vi "Test Executive.vi"(11 "Module Config":T30={"Name"="Test Executive", "Parent Q"=refnum, "Is Child?"=FALSE, "Index"=0, "Dirs"={"Root"=path "C:/MTE", "Config"=path "C:/MTE/Config", "Logs"=path "C:/MTE/Logs", "Reports"=path "C:/ATE/Reports", "App Data"=path "C:/ProgramData/Test Executive"}, "Simulate"=FALSE, "SimCtrl"=refnum}) -> ()   [LabVIEW 2018] (continued)
          frame "Repeat Sequence", "Repeat Sequence - Auto" {
            n805 = call <vilib>:"Scheduler.Delete Task.vi"("Sched Name"="Repeat Notification", "Q In"=w1672) -> ("Q Out"=w1671:refnum<queue>)  [unwired: 8 in, 1 out]
            n806 = Flush Queue(queue=w1671) -> (queue out=w1670:refnum<queue>)  [unwired: 1 in, 2 out]
            n807 = Bundle By Name(cluster=w1676, "Opts.NotValOper"=FALSE ("Opts.ClearSN")) -> (w1675:T73)
            n808 = property on="Repeat Notificaiton" class="Str"("Visible"=FALSE) -> ()  [unwired: 2 in, 2 out]
            n809 = call <vilib>:"Q.Enqueue Seq.vi"("Seq Task Name"="Test Reset" ("Task Name"), "Q In"=w1670) -> ("Q Out"=w1677:refnum<queue>)  [unwired: 8 in, 1 out]
            n810 = call <vilib>:"Q.Enqueue Seq.vi"("Seq Task Name"="Test Start", "Q In"=w1677) -> ()  [unwired: 8 in, 2 out]
            n811 = property on="Kill AutoLnch" class="Bool"("Visible"=FALSE) -> ()  [unwired: 2 in, 2 out]
          }
          frame "Request Vars" {
            n812 = Bundle By Name(cluster=w1682, "Lists.ReqVars"=TRUE) -> (w1683:T73)
          }
          frame "Result - Attributes" {
            w1700 = T43[] []  # Attr
            # "Result - Attributes(1D Array of Attribute)"
            n813 = Variant To Data(type=w1700, Variant=w1686) -> (data=w1688:T43[], error out=w1685:errorcluster)  [unwired: 1 in]
            n814 = case shown="Error" w1685 {
              tunnel: w1686 -> [_ w1708]
              tunnel: w1688 -> [w1704 _]
              tunnel: [w1704 w1705] -> w1687
              frame No Error {
              }
              frame Error {
                n815 = Variant To Data(type=T44[] [], Variant=w1708) -> (data=w1706:T44[])  [unwired: 1 in, 1 out]
                n816 = call "Result.Attribute, Convert EV1 to EV2 Format.vi"("Attr EV1"=w1706) -> ("Attr EV2"=w1705:T43[])  [unwired: 10 in]
              }
            }
            n817 = Unbundle By Name(w1701) -> ("ResultState"=w1692:T63, "SectCtr"=w1699:T72, "Data.Meas"=w1696:T38[], "Lists.Limits"=w1695:variant)
            n818 = call <vilib>:"Q.Enqueue Task.vi"("Top of Q"=TRUE, "Task Name"="Update Result Table", "Q In"=w1689) -> ()  [unwired: 7 in, 2 out]
            n819 = for {
              tunnel: w1687 -> [w1710] mode=indexing
              shift-right: [w1717] -> w1698
              shift-left: w1699 -> [w1718]
              tunnel: [w1715] -> w1697 mode=indexing
              tunnel: w1695 -> [w1711]
              n820 = call "Result.Attribute, Convert V2 to Measurement V1 Format.vi"("Attribute"=w1710) -> ("Meas"=w1709:T38)  [unwired: 10 in]
              n821 = call "Result.Measurement Look Up Limits.vi"("Meas"=w1709, "Limits"=w1711) -> ("Measurement Out"=w1712:T38)  [unwired: 4 in]
              n822 = call "Step Counter.Step Count Controller.vi"("Step Action"=Step_Counter.Action."Data +", "Step State"=w1718) -> ("Step"=w1716:string, "Step State Out"=w1717:T72, "Cntr"=w1713:i32)  [unwired: 7 in]
              n823 = Bundle By Name(cluster=w1712, "Step"=w1716, "Cnt"=w1713) -> (w1715:T38)
            }
            n824 = Build Array (concatenate)(w1696, w1697) -> (w1693:T38[])
            n825 = call "Result.Measurement, Screen for Fail or Error.vi"("Num"=w1693, "ResultState In"=w1692) -> ("ResultState Out"=w1694:T63)  [unwired: 9 in]
            n826 = Bundle By Name(cluster=w1701, "ResultState"=w1694, "SectCtr"=w1698, "Data.Meas"=w1693) -> (w1702:T73)
          }
          frame "Result - File Objs" {
            n827 = Variant To Data(type=T29[] [] ("File Data Objs"), Variant=w1726) -> (data=w1727:T29[])  [unwired: 1 in, 1 out]
            n828 = Unbundle By Name(w1720) -> ("Cfg.Dirs.Reports"=w1722:path)
            n829 = Unbundle By Name(w1737) -> ("SectCtr"=w1736:T72, "Data.FileObjs"=w1733:T29[], "Lists.Limits"=w1732:variant)
            n830 = call <vilib>:"Q.Enqueue Task.vi"("Top of Q"=TRUE, "Task Name"="Update Result Table", "Q In"=w1728) -> ()  [unwired: 7 in, 2 out]
            n831 = Build Path(base path=w1722, name or relative path="Current Test Data Files") -> (appended path=w1719:path)
            n832 = for {
              tunnel: w1727 -> [w1747] mode=indexing
              shift-right: [w1752] -> w1735
              shift-left: w1736 -> [w1753]
              tunnel: [w1750] -> w1734 mode=indexing
              tunnel: w1732 -> [_]
              tunnel: [w1740] -> w1724 mode=indexing
              tunnel: w1719 -> [w1739]
              n833 = Unbundle By Name(w1747) -> ("Path"=w1743:path)
              n834 = Strip Path(path=w1743) -> (name=w1742:string)  [unwired: 1 out]
              n835 = call "Step Counter.Step Count Controller.vi"("Step Action"=Step_Counter.Action."Data +", "Step State"=w1753) -> ("Step"=w1751:string, "Step State Out"=w1752:T72, "Cntr"=w1748:i32)  [unwired: 7 in]
              n836 = Build Path(base path=w1739, name or relative path=w1742) -> (appended path=w1741:path)
              n837 = call "File.Move_Copy File, Overwrite if Exists.vi"("Move(F)/Copy(T)"=TRUE, "SkipIfExists(F)/Overwrite(T)"=TRUE, "Target Path"=w1741, "Source Path"=w1743) -> ("error out"=w1740:errorcluster, "Target Out"=w1744:path)  [unwired: 6 in]
              n838 = Bundle By Name(cluster=w1747, "Step"=w1751, "Cnt"=w1748, "Path"=w1744) -> (w1750:T29)
            }
            n839 = Merge Errors(w1724) -> (w1723:errorcluster)
            n840 = Build Array (concatenate)(w1733, w1734) -> (w1731:T29[])
            n841 = Bundle By Name(cluster=w1737, "SectCtr"=w1735, "Data.FileObjs"=w1731) -> (w1738:T73)
          }
          frame "Result - Reports" {
            n842 = local read "Seq Rslt"() -> (w1754:string)
            n843 = Unbundle By Name(w1758) -> ("RptCfg"=w1759:T17[])
            n844 = for {
              tunnel: w1759 -> [w1767] mode=indexing
              tunnel: w1758 -> [w1765]
              tunnel: w1757 -> [w1763]
              tunnel: [w1764] -> w1755 mode=indexing
              tunnel: w1754 -> [w1761]
              n845 = Unbundle By Name(w1767) -> ("Type"=w1766:T18, "Seq_Dir"=w1762:cluster{"Sequence":string, "Folder":path}[])
              n846 = call "TestExec.Configure Reports, Lookup Rpt Dir.vi"("Seq Name"=w1761, "Seq_Dir"=w1762) -> ("Folder"=w1760:path)  [unwired: 9 in]
              n847 = case shown="\"XLINK_ResultOnly\"" w1766 {
                tunnel: w1765 -> [w1778 w1809 w1839 w1870 w1900 w1938]
                tunnel: [w1775 w1806 w1836 w1867 w1897 w1935] -> w1764
                tunnel: w1763 -> [_ _ _ _ _ w1926]
                tunnel: w1760 -> [w1768 w1798 w1829 w1859 w1890 w1920]
                frame "CSV", Default {
                  n848 = Unbundle By Name(w1778) -> ("RptHdr"=w1790:T70, "RptUUT"=w1792:T50, "Data.Meas"=w1789:T38[], "ResultState"=w1783:T63)
                  n849 = Unbundle By Name(w1783) -> ("Code"=w1782:i32, "Description"=w1781:string, "State"=w1780:T1)
                  n850 = call <vilib>:"File.Create Folder if Does Not Exist.vi"("Path"=w1768) -> ("error out"=w1772:errorcluster, "Dup Path"=w1771:path)  [unwired: 8 in, 1 out]
                  n851 = case shown="\"None\", Default" w1780 {
                    tunnel: [TestResult.Symptom.State."Completed" ("Result.Result") TestResult.Symptom.State."Pass" ("Result.Result") TestResult.Symptom.State."Fail" ("Result.Result") TestResult.Symptom.State."Aborted" ("Result.Result") TestResult.Symptom.State."Error" ("Result.Result")] -> w1779
                    frame "None", Default {
                    }
                    frame "Passing", "PASS" {
                    }
                    frame "Failing", "FAIL" {
                    }
                    frame "ABORT" {
                    }
                    frame "ERROR" {
                    }
                  }
                  n852 = Bundle By Name(cluster=w1792, "Measurements.Measurement"=w1789, "Result.Code"=w1782, "Result.Description"=w1781, "Result.Result"=w1779) -> (w1785:T50)
                  n853 = Format Into String(format string="Error creating report folder \"%s\".", w1771) -> (resulting string=w1773:string)  [unwired: 2 in, 1 out]
                  n854 = Unbundle By Name(w1790) -> ("Station"=w1788:T47, "Test Run"=w1787:T48, "Test Sequence"=w1786:T49)  [unwired: 1 out]
                  n855 = call "Error.Set-Change Error Info.vi"("Append Details"=FALSE, "error in"=w1772, "Description"=w1773) -> ("error out"=w1770:errorcluster)  [unwired: 8 in]
                  n856 = Build Array(w1785) -> (w1784:T50[])
                  n857 = Bundle By Name(cluster=T46 {"#attributes"={"Version"="MTE_1.0.0"}, "Station"={"Name"="", "PN"="", "SN"="", "Rev"="", "PC Name"="", "Location"="", "HW_Config"={"HW_Item"=[]}, "SW_Config"={"SW_Item"=[]}}, "Test Run"={"Operator"="", "Start Time"=timestamp(0 s since 1904-01-01), "Duration(s)"=0.0, "Mode"="", "Comment"="", "ProcessStep"=""}, "Test Sequence"={"Name"="", "Config"={"Config_Item"=[]}}, "UUTs"={"UUT"=[]}} ("Test Result"), "Station"=w1788, "Test Run"=w1787, "Test Sequence"=w1786, "UUTs.UUT"=w1784) -> (w1776:T46)
                  n858 = call "Result.Report Creator.vi"("error in"=w1770, "Data"=w1776, "Format"=Result.Report_Format_Selector."CSV", "OutputDir"=w1771) -> ("error out"=w1775:errorcluster)  [unwired: 6 in, 1 out]
                }
                frame "CSV_SummaryResult" {
                  n859 = Unbundle By Name(w1809) -> ("RptHdr"=w1821:T70, "RptUUT"=w1823:T50, "Data.Meas"=w1820:T38[], "ResultState"=w1814:T63)
                  n860 = Unbundle By Name(w1814) -> ("Code"=w1813:i32, "Description"=w1812:string, "State"=w1811:T1)
                  n861 = call <vilib>:"File.Create Folder if Does Not Exist.vi"("Path"=w1798) -> ("error out"=w1803:errorcluster, "Dup Path"=w1802:path)  [unwired: 8 in, 1 out]
                  n862 = case shown="\"None\", Default" w1811 {
                    tunnel: [TestResult.Symptom.State."Completed" ("Result.Result") TestResult.Symptom.State."Pass" ("Result.Result") TestResult.Symptom.State."Fail" ("Result.Result") TestResult.Symptom.State."Aborted" ("Result.Result") TestResult.Symptom.State."Error" ("Result.Result")] -> w1810
                    frame "None", Default {
                    }
                    frame "Passing", "PASS" {
                    }
                    frame "Failing", "FAIL" {
                    }
                    frame "ABORT" {
                    }
                    frame "ERROR" {
                    }
                  }
                  n863 = Bundle By Name(cluster=w1823, "Measurements.Measurement"=w1820, "Result.Code"=w1813, "Result.Description"=w1812, "Result.Result"=w1810) -> (w1816:T50)
                  n864 = Format Into String(format string="Error creating report folder \"%s\".", w1802) -> (resulting string=w1804:string)  [unwired: 2 in, 1 out]
                  n865 = Unbundle By Name(w1821) -> ("Station"=w1819:T47, "Test Run"=w1818:T48, "Test Sequence"=w1817:T49)  [unwired: 1 out]
                  n866 = call "Error.Set-Change Error Info.vi"("Append Details"=FALSE, "error in"=w1803, "Description"=w1804) -> ("error out"=w1801:errorcluster)  [unwired: 8 in]
                  n867 = Build Array(w1816) -> (w1815:T50[])
                  n868 = Bundle By Name(cluster=T46 {"#attributes"={"Version"="MTE_1.0.0"}, "Station"={"Name"="", "PN"="", "SN"="", "Rev"="", "PC Name"="", "Location"="", "HW_Config"={"HW_Item"=[]}, "SW_Config"={"SW_Item"=[]}}, "Test Run"={"Operator"="", "Start Time"=timestamp(0 s since 1904-01-01), "Duration(s)"=0.0, "Mode"="", "Comment"="", "ProcessStep"=""}, "Test Sequence"={"Name"="", "Config"={"Config_Item"=[]}}, "UUTs"={"UUT"=[]}} ("Test Result"), "Station"=w1819, "Test Run"=w1818, "Test Sequence"=w1817, "UUTs.UUT"=w1815) -> (w1807:T46)
                  n869 = call "Result.Report Creator.vi"("PassFailResultOnly"=TRUE ("Xlink Overall Result Only"), "error in"=w1801, "Data"=w1807, "Format"=Result.Report_Format_Selector."CSV", "OutputDir"=w1802) -> ("error out"=w1806:errorcluster)  [unwired: 5 in, 1 out]
                }
                frame "XLINK" {
                  n870 = Unbundle By Name(w1839) -> ("RptHdr"=w1851:T70, "RptUUT"=w1853:T50, "Data.Meas"=w1850:T38[], "ResultState"=w1844:T63)
                  n871 = Unbundle By Name(w1844) -> ("Code"=w1843:i32, "Description"=w1842:string, "State"=w1841:T1)
                  n872 = call <vilib>:"File.Create Folder if Does Not Exist.vi"("Path"=w1829) -> ("error out"=w1833:errorcluster, "Dup Path"=w1832:path)  [unwired: 8 in, 1 out]
                  n873 = case shown="\"None\", Default" w1841 {
                    tunnel: [TestResult.Symptom.State."Completed" ("Result.Result") TestResult.Symptom.State."Pass" ("Result.Result") TestResult.Symptom.State."Fail" ("Result.Result") TestResult.Symptom.State."Aborted" ("Result.Result") TestResult.Symptom.State."Error" ("Result.Result")] -> w1840
                    frame "None", Default {
                    }
                    frame "Passing", "PASS" {
                    }
                    frame "Failing", "FAIL" {
                    }
                    frame "ABORT" {
                    }
                    frame "ERROR" {
                    }
                  }
                  n874 = Bundle By Name(cluster=w1853, "Measurements.Measurement"=w1850, "Result.Code"=w1843, "Result.Description"=w1842, "Result.Result"=w1840) -> (w1846:T50)
                  n875 = Format Into String(format string="Error creating report folder \"%s\".", w1832) -> (resulting string=w1834:string)  [unwired: 2 in, 1 out]
                  n876 = Unbundle By Name(w1851) -> ("Station"=w1849:T47, "Test Run"=w1848:T48, "Test Sequence"=w1847:T49)  [unwired: 1 out]
                  n877 = call "Error.Set-Change Error Info.vi"("Append Details"=FALSE, "error in"=w1833, "Description"=w1834) -> ("error out"=w1831:errorcluster)  [unwired: 8 in]
                  n878 = Build Array(w1846) -> (w1845:T50[])
                  n879 = Bundle By Name(cluster=T46 {"#attributes"={"Version"="MTE_1.0.0"}, "Station"={"Name"="", "PN"="", "SN"="", "Rev"="", "PC Name"="", "Location"="", "HW_Config"={"HW_Item"=[]}, "SW_Config"={"SW_Item"=[]}}, "Test Run"={"Operator"="", "Start Time"=timestamp(0 s since 1904-01-01), "Duration(s)"=0.0, "Mode"="", "Comment"="", "ProcessStep"=""}, "Test Sequence"={"Name"="", "Config"={"Config_Item"=[]}}, "UUTs"={"UUT"=[]}} ("Test Result"), "Station"=w1849, "Test Run"=w1848, "Test Sequence"=w1847, "UUTs.UUT"=w1845) -> (w1837:T46)
                  n880 = call "Result.Report Creator.vi"("error in"=w1831, "Data"=w1837, "Format"=Result.Report_Format_Selector."Xlink XML", "OutputDir"=w1832) -> ("error out"=w1836:errorcluster)  [unwired: 6 in, 1 out]
                }
                frame "XLINK_ResultOnly" {
                  n881 = Unbundle By Name(w1870) -> ("RptHdr"=w1882:T70, "RptUUT"=w1884:T50, "Data.Meas"=w1881:T38[], "ResultState"=w1875:T63)
                  n882 = Unbundle By Name(w1875) -> ("Code"=w1874:i32, "Description"=w1873:string, "State"=w1872:T1)
                  n883 = call <vilib>:"File.Create Folder if Does Not Exist.vi"("Path"=w1859) -> ("error out"=w1864:errorcluster, "Dup Path"=w1863:path)  [unwired: 8 in, 1 out]
                  n884 = case shown="\"None\", Default" w1872 {
                    tunnel: [TestResult.Symptom.State."Completed" ("Result.Result") TestResult.Symptom.State."Pass" ("Result.Result") TestResult.Symptom.State."Fail" ("Result.Result") TestResult.Symptom.State."Aborted" ("Result.Result") TestResult.Symptom.State."Error" ("Result.Result")] -> w1871
                    frame "None", Default {
                    }
                    frame "Passing", "PASS" {
                    }
                    frame "Failing", "FAIL" {
                    }
                    frame "ABORT" {
                    }
                    frame "ERROR" {
                    }
                  }
                  n885 = Bundle By Name(cluster=w1884, "Measurements.Measurement"=w1881, "Result.Code"=w1874, "Result.Description"=w1873, "Result.Result"=w1871) -> (w1877:T50)
                  n886 = Format Into String(format string="Error creating report folder \"%s\".", w1863) -> (resulting string=w1865:string)  [unwired: 2 in, 1 out]
                  n887 = Unbundle By Name(w1882) -> ("Station"=w1880:T47, "Test Run"=w1879:T48, "Test Sequence"=w1878:T49)  [unwired: 1 out]
                  n888 = call "Error.Set-Change Error Info.vi"("Append Details"=FALSE, "error in"=w1864, "Description"=w1865) -> ("error out"=w1862:errorcluster)  [unwired: 8 in]
                  n889 = Build Array(w1877) -> (w1876:T50[])
                  n890 = Bundle By Name(cluster=T46 {"#attributes"={"Version"="MTE_1.0.0"}, "Station"={"Name"="", "PN"="", "SN"="", "Rev"="", "PC Name"="", "Location"="", "HW_Config"={"HW_Item"=[]}, "SW_Config"={"SW_Item"=[]}}, "Test Run"={"Operator"="", "Start Time"=timestamp(0 s since 1904-01-01), "Duration(s)"=0.0, "Mode"="", "Comment"="", "ProcessStep"=""}, "Test Sequence"={"Name"="", "Config"={"Config_Item"=[]}}, "UUTs"={"UUT"=[]}} ("Test Result"), "Station"=w1880, "Test Run"=w1879, "Test Sequence"=w1878, "UUTs.UUT"=w1876) -> (w1868:T46)
                  n891 = call "Result.Report Creator.vi"("PassFailResultOnly"=TRUE, "error in"=w1862, "Data"=w1868, "Format"=Result.Report_Format_Selector."Xlink XML", "OutputDir"=w1863) -> ("error out"=w1867:errorcluster)  [unwired: 5 in, 1 out]
                }
                frame "JSON" {
                  n892 = Unbundle By Name(w1900) -> ("RptHdr"=w1912:T70, "RptUUT"=w1914:T50, "Data.Meas"=w1911:T38[], "ResultState"=w1905:T63)
                  n893 = Unbundle By Name(w1905) -> ("Code"=w1904:i32, "Description"=w1903:string, "State"=w1902:T1)
                  n894 = case shown="\"None\", Default" w1902 {
                    tunnel: [TestResult.Symptom.State."Completed" ("Result.Result") TestResult.Symptom.State."Pass" ("Result.Result") TestResult.Symptom.State."Fail" ("Result.Result") TestResult.Symptom.State."Aborted" ("Result.Result") TestResult.Symptom.State."Error" ("Result.Result")] -> w1901
                    frame "None", Default {
                    }
                    frame "Passing", "PASS" {
                    }
                    frame "Failing", "FAIL" {
                    }
                    frame "ABORT" {
                    }
                    frame "ERROR" {
                    }
                  }
                  n895 = call <vilib>:"File.Create Folder if Does Not Exist.vi"("Path"=w1890) -> ("error out"=w1892:errorcluster, "Dup Path"=w1895:path)  [unwired: 8 in, 1 out]
                  n896 = Bundle By Name(cluster=w1914, "Measurements.Measurement"=w1911, "Result.Code"=w1904, "Result.Description"=w1903, "Result.Result"=w1901) -> (w1907:T50)
                  n897 = Unbundle By Name(w1912) -> ("Station"=w1910:T47, "Test Run"=w1909:T48, "Test Sequence"=w1908:T49)  [unwired: 1 out]
                  n898 = Format Into String(format string="Error creating report folder \"%s\".", w1895) -> (resulting string=w1894:string)  [unwired: 2 in, 1 out]
                  n899 = Build Array(w1907) -> (w1906:T50[])
                  n900 = call "Error.Set-Change Error Info.vi"("Append Details"=FALSE, "error in"=w1892, "Description"=w1894) -> ("error out"=w1893:errorcluster)  [unwired: 8 in]
                  n901 = Bundle By Name(cluster=T46 {"#attributes"={"Version"="MTE_1.0.0"}, "Station"={"Name"="", "PN"="", "SN"="", "Rev"="", "PC Name"="", "Location"="", "HW_Config"={"HW_Item"=[]}, "SW_Config"={"SW_Item"=[]}}, "Test Run"={"Operator"="", "Start Time"=timestamp(0 s since 1904-01-01), "Duration(s)"=0.0, "Mode"="", "Comment"="", "ProcessStep"=""}, "Test Sequence"={"Name"="", "Config"={"Config_Item"=[]}}, "UUTs"={"UUT"=[]}} ("Test Result"), "Station"=w1910, "Test Run"=w1909, "Test Sequence"=w1908, "UUTs.UUT"=w1906) -> (w1898:T46)
                  n902 = call "Result.Report Creator.vi"("error in"=w1893, "Data"=w1898, "Format"=Result.Report_Format_Selector."JSON", "OutputDir"=w1895) -> ("error out"=w1897:errorcluster)  [unwired: 6 in, 1 out]
                }
                frame "JSON_WithFiles" {
                  n903 = Unbundle By Name(w1938) -> ("RptHdr"=w1950:T70, "RptUUT"=w1952:T50, "Data.Meas"=w1949:T38[], "ResultState"=w1943:T63, "Data.FileObjs"=w1930:T29[])
                  n904 = Unbundle By Name(w1926) -> ("Cfg.Dirs.Reports"=w1928:path)
                  n905 = Unbundle By Name(w1943) -> ("Code"=w1942:i32, "Description"=w1941:string, "State"=w1940:T1)
                  n906 = Build Path(base path=w1928, name or relative path="Temp Results") -> (appended path=w1929:path)
                  n907 = case shown="\"None\", Default" w1940 {
                    tunnel: [TestResult.Symptom.State."Completed" ("Result.Result") TestResult.Symptom.State."Pass" ("Result.Result") TestResult.Symptom.State."Fail" ("Result.Result") TestResult.Symptom.State."Aborted" ("Result.Result") TestResult.Symptom.State."Error" ("Result.Result")] -> w1939
                    frame "None", Default {
                    }
                    frame "Passing", "PASS" {
                    }
                    frame "Failing", "FAIL" {
                    }
                    frame "ABORT" {
                    }
                    frame "ERROR" {
                    }
                  }
                  n908 = call <vilib>:"File.Create Folder if Does Not Exist.vi"("Path"=w1920) -> ("error out"=w1923:errorcluster, "Dup Path"=w1933:path)  [unwired: 8 in, 1 out]
                  n909 = call <vilib>:"File.Create Folder if Does Not Exist.vi"("Path"=w1929) -> ("error out"=w1924:errorcluster, "Dup Path"=w1925:path)  [unwired: 8 in, 1 out]
                  n910 = Bundle By Name(cluster=w1952, "Measurements.Measurement"=w1949, "Result.Code"=w1942, "Result.Description"=w1941, "Result.Result"=w1939) -> (w1945:T50)
                  n911 = Merge Errors(w1924, w1923) -> (w1922:errorcluster)
                  n912 = Unbundle By Name(w1950) -> ("Station"=w1948:T47, "Test Run"=w1947:T48, "Test Sequence"=w1946:T49)  [unwired: 1 out]
                  n913 = Format Into String(format string="Error creating report folder \"%s\".", w1933) -> (resulting string=w1932:string)  [unwired: 2 in, 1 out]
                  n914 = Build Array(w1945) -> (w1944:T50[])
                  n915 = call "Error.Set-Change Error Info.vi"("Append Details"=FALSE, "error in"=w1922, "Description"=w1932) -> ("error out"=w1931:errorcluster)  [unwired: 8 in]
                  n916 = Bundle By Name(cluster=T46 {"#attributes"={"Version"="MTE_1.0.0"}, "Station"={"Name"="", "PN"="", "SN"="", "Rev"="", "PC Name"="", "Location"="", "HW_Config"={"HW_Item"=[]}, "SW_Config"={"SW_Item"=[]}}, "Test Run"={"Operator"="", "Start Time"=timestamp(0 s since 1904-01-01), "Duration(s)"=0.0, "Mode"="", "Comment"="", "ProcessStep"=""}, "Test Sequence"={"Name"="", "Config"={"Config_Item"=[]}}, "UUTs"={"UUT"=[]}} ("Test Result"), "Station"=w1948, "Test Run"=w1947, "Test Sequence"=w1946, "UUTs.UUT"=w1944) -> (w1936:T46)
                  n917 = call "Result.Report Creator.vi"("Temp Folder"=w1925, "File Data Objs"=w1930, "error in"=w1931, "Data"=w1936, "Format"=Result.Report_Format_Selector."JSON with Files", "OutputDir"=w1933) -> ("error out"=w1935:errorcluster)  [unwired: 4 in, 1 out]
                }
              }
            }
            n918 = Merge Errors(w1755) -> (w1756:errorcluster)
          }
          frame "Result - CSV Report" {
            # "Obsolete - Remove"
            n919 = Variant To Data(type=FALSE, Variant=w1962) -> (data=w1959:bool, error out=w1960:errorcluster)  [unwired: 1 in]
            n920 = Unbundle By Name(w1972) -> ("RptHdr"=w1984:T70, "RptUUT"=w1986:T50, "Data.Meas"=w1983:T38[], "ResultState"=w1977:T63)
            n921 = Unbundle By Name(w1977) -> ("Code"=w1976:i32, "Description"=w1975:string, "State"=w1974:T1)
            n922 = call <vilib>:"Clear Errors.vi"("error in (no error)"=w1960) -> ()  [unwired: 5 in, 2 out]
            n923 = case shown="\"None\", Default" w1974 {
              tunnel: [TestResult.Symptom.State."Completed" ("Result.Result") TestResult.Symptom.State."Pass" ("Result.Result") TestResult.Symptom.State."Fail" ("Result.Result") TestResult.Symptom.State."Aborted" ("Result.Result") TestResult.Symptom.State."Error" ("Result.Result")] -> w1973
              frame "None", Default {
              }
              frame "Passing", "PASS" {
              }
              frame "Failing", "FAIL" {
              }
              frame "ABORT" {
              }
              frame "ERROR" {
              }
            }
            n924 = Unbundle By Name(w1970) -> ("Cfg.Dirs.Reports"=w1969:path)
            n925 = Bundle By Name(cluster=w1986, "Measurements.Measurement"=w1983, "Result.Code"=w1976, "Result.Description"=w1975, "Result.Result"=w1973) -> (w1979:T50)
            n926 = Build Path(base path=w1969, name or relative path="CSV") -> (appended path=w1967:path)
            n927 = Unbundle By Name(w1984) -> ("Station"=w1982:T47, "Test Run"=w1981:T48, "Test Sequence"=w1980:T49)  [unwired: 1 out]
            n928 = call <vilib>:"File.Create Folder if Does Not Exist.vi"("Path"=w1967) -> ("error out"=w1965:errorcluster, "Dup Path"=w1966:path)  [unwired: 8 in, 1 out]
            n929 = Build Array(w1979) -> (w1978:T50[])
            n930 = Bundle By Name(cluster=T46 {"#attributes"={"Version"="MTE_1.0.0"}, "Station"={"Name"="", "PN"="", "SN"="", "Rev"="", "PC Name"="", "Location"="", "HW_Config"={"HW_Item"=[]}, "SW_Config"={"SW_Item"=[]}}, "Test Run"={"Operator"="", "Start Time"=timestamp(0 s since 1904-01-01), "Duration(s)"=0.0, "Mode"="", "Comment"="", "ProcessStep"=""}, "Test Sequence"={"Name"="", "Config"={"Config_Item"=[]}}, "UUTs"={"UUT"=[]}} ("Test Result"), "Station"=w1982, "Test Run"=w1981, "Test Sequence"=w1980, "UUTs.UUT"=w1978) -> (w1971:T46)
            n931 = call "Result.Report Creator.vi"("error in"=w1965, "Data"=w1971, "Format"=Result.Report_Format_Selector."CSV", "OutputDir"=w1966) -> ("error out"=w1964:errorcluster, "Output File"=w1958:path)  [unwired: 6 in]
            n932 = case shown="True" w1959 {
              tunnel: w1964 -> [w1988 w1991]
              tunnel: [w1988 w1990] -> w1963
              tunnel: w1958 -> [_ w1989]
              frame False {
              }
              frame True {
                n933 = call <vilib>:"File.Open File or Folder.vi"("Error In"=w1991, "Path"=w1989) -> ("Error Out"=w1990:errorcluster)  [unwired: 9 in]
              }
            }
          }
          frame "Result - Error" {
            # "Result - Error(Error Cluster)"
            n934 = Variant To Data(type=errorcluster {"status"=FALSE, "code"=0, "source"=""} ("error constant"), Variant=w2001) -> (data=w1997:errorcluster)  [unwired: 1 in, 1 out]
            n935 = Bundle By Name(cluster=w1999, "ResultError"=w1997) -> (w1998:T73)
          }
          frame "Result - Measurements", "Result - Numeric" {
            w2007 = T74 -6000 items=["No Error"=0, "Abort"=-2, "Misc"=-5000, "Fixture Error"=-5100, "File IO - General"=-5200, "FIle IO - Config Error"=-5201, "Instrument - General"=-5300, "Instrument - Serial Com"=-5301, "Instrument - Camera"=-5302, "Instrument - PS"=-5303, "Instrument - Oscilloscope"=-5304, "Instrument - Function Gen"=-5305, "Instrument - Load"=-5306, "Instrument - Meter"=-5307, "Instrument - Power Control"=-5308, "Instrument - Motion"=-5309, "Instrument - RF"=-5310, "System Exe"=-5400, "Image Processing"=-5500, "Communication"=-5600, "Script - Syntax Error"=-6000, "Script - Invalid Name or Param"=-6100, "Script - Timeout"=-6200, "Invalid Data"=-6300, "FW Update Error"=-6500] ("Std Code")
            n936 = for {
              N: 3 -> [_]
              tunnel: w2006 -> [w2026]
              tunnel: [w2025] -> w2005
              tunnel: [w2024] -> w2004
              i -> [w2027]
              stop <- w2024 continue-if-true
              n937 = case shown="0, Default" w2027 {
                tunnel: [w2028 w2035 w2041] -> w2024
                tunnel: w2026 -> [w2031 w2034 w2040]
                tunnel: [w2029 w2033 w2039] -> w2025
                frame 0, Default {
                  n938 = Variant To Data(type=T38[] [], Variant=w2031) -> (data=w2029:T38[], error out=w2028:errorcluster)  [unwired: 1 in]
                }
                frame 1 {
                  w2036 = T77[] []  # Num
                  n939 = Variant To Data(type=w2036, Variant=w2034) -> (data=w2032:T77[], error out=w2035:errorcluster)  [unwired: 1 in]
                  n940 = call "Result.Numeric, Array, Convert V2 to Measurement V1 Format.vi"("Num In"=w2032) -> ("Meas Out"=w2033:T38[])  [unwired: 10 in]
                }
                frame 2 {
                  w2042 = T78[] []  # Num
                  n941 = Variant To Data(type=w2042, Variant=w2040) -> (data=w2038:T78[], error out=w2041:errorcluster)  [unwired: 1 in]
                  n942 = call "Result.Numeric, Convert EV1 to EV2 Format.vi"("Num EV1"=w2038) -> ("Num EV2"=w2037:T77[])  [unwired: 10 in]
                  n943 = call "Result.Numeric, Array, Convert V2 to Measurement V1 Format.vi"("Num In"=w2037) -> ("Meas Out"=w2039:T38[])  [unwired: 10 in]
                }
              }
            }
            n944 = Unbundle By Name(w2018) -> ("ResultState"=w2013:T63, "SectCtr"=w2020:T72, "Data.Meas"=w2022:T38[], "Lists.Limits"=w2016:variant)
            n945 = call <vilib>:"Q.Enqueue Task.vi"("Top of Q"=TRUE, "Task Name"="Update Result Table", "Q In"=w2012) -> ()  [unwired: 7 in, 2 out]
            n946 = for {
              tunnel: w2005 -> [w2043] mode=indexing
              shift-right: [w2050] -> w2021
              shift-left: w2020 -> [w2051]
              tunnel: [w2048] -> w2019 mode=indexing
              tunnel: w2016 -> [w2044]
              n947 = call "Result.Measurement Look Up Limits.vi"("Meas"=w2043, "Limits"=w2044) -> ("Measurement Out"=w2045:T38)  [unwired: 4 in]
              n948 = call "Step Counter.Step Count Controller.vi"("Step Action"=Step_Counter.Action."Data +", "Step State"=w2051) -> ("Step"=w2049:string, "Step State Out"=w2050:T72, "Cntr"=w2046:i32)  [unwired: 7 in]
              n949 = Bundle By Name(cluster=w2045, "Step"=w2049, "Cnt"=w2046) -> (w2048:T38)
            }
            n950 = call "Error.Set-Change Error Info.vi"("Std Code"=w2007, "error in"=w2004, "Description"="Invalid data type used for \"Result - Measurements\".") -> ("error out"=w2003:errorcluster)  [unwired: 8 in]
            n951 = Build Array (concatenate)(w2022, w2019) -> (w2015:T38[])
            n952 = call "Result.Measurement, Screen for Fail or Error.vi"("Num"=w2015, "ResultState In"=w2013) -> ("ResultState Out"=w2014:T63)  [unwired: 9 in]
            n953 = Bundle By Name(cluster=w2018, "ResultState"=w2014, "SectCtr"=w2021, "Data.Meas"=w2015) -> (w2017:T73)
          }
          frame "Result - Overwrite Attribute Data" {
            w2057 = T43[] []  # Attr
            # "Result - Over Write Attr Data(1D Array of Attribute)"
            n954 = Variant To Data(type=w2057, Variant=w2054) -> (data=w2056:T43[], error out=w2055:errorcluster)  [unwired: 1 in]
            n955 = call <vilib>:"Q.Enqueue Task.vi"("Top of Q"=TRUE, "Task Name"="Update Result Table", "Q In"=w2058) -> ()  [unwired: 7 in, 2 out]
            n956 = case shown="Error" w2055 {
              tunnel: w2054 -> [_ w2070]
              tunnel: w2056 -> [w2066 _]
              tunnel: [w2066 w2067] -> w2053
              frame No Error {
              }
              frame Error {
                n957 = Variant To Data(type=T44[] [], Variant=w2070) -> (data=w2068:T44[])  [unwired: 1 in, 1 out]
                n958 = call "Result.Attribute, Convert EV1 to EV2 Format.vi"("Attr EV1"=w2068) -> ("Attr EV2"=w2067:T43[])  [unwired: 10 in]
              }
            }
            n959 = for {
              tunnel: w2053 -> [w2065] mode=indexing
              tunnel: [w2064] -> w2052 mode=indexing
              n960 = call "Result.Attribute, Convert V2 to Measurement V1 Format.vi"("Attribute"=w2065) -> ("Meas"=w2064:T38)  [unwired: 10 in]
            }
            n961 = Bundle By Name(cluster=w2061, "Data.Meas"=w2052) -> (w2062:T73)
          }
          frame "Result - Overwrite Measurement Data", "Result - Overwrite Numeric Data" {
            # "Result - Over Write Numeric Data(1D Array of Num Result)"
            n962 = for {
              N: 3 -> [_]
              tunnel: w2072 -> [w2082]
              tunnel: [w2081] -> w2071
              tunnel: [w2080] -> _
              i -> [w2083]
              stop <- w2080 continue-if-true
              n963 = case shown="0, Default" w2083 {
                tunnel: [w2084 w2091 w2097] -> w2080
                tunnel: w2082 -> [w2087 w2090 w2096]
                tunnel: [w2085 w2089 w2095] -> w2081
                frame 0, Default {
                  n964 = Variant To Data(type=T38[] [], Variant=w2087) -> (data=w2085:T38[], error out=w2084:errorcluster)  [unwired: 1 in]
                }
                frame 1 {
                  w2092 = T77[] []  # Num
                  n965 = Variant To Data(type=w2092, Variant=w2090) -> (data=w2088:T77[], error out=w2091:errorcluster)  [unwired: 1 in]
                  n966 = call "Result.Numeric, Array, Convert V2 to Measurement V1 Format.vi"("Num In"=w2088) -> ("Meas Out"=w2089:T38[])  [unwired: 10 in]
                }
                frame 2 {
                  w2098 = T78[] []  # Num
                  n967 = Variant To Data(type=w2098, Variant=w2096) -> (data=w2094:T78[], error out=w2097:errorcluster)  [unwired: 1 in]
                  n968 = call "Result.Numeric, Convert EV1 to EV2 Format.vi"("Num EV1"=w2094) -> ("Num EV2"=w2093:T77[])  [unwired: 10 in]
                  n969 = call "Result.Numeric, Array, Convert V2 to Measurement V1 Format.vi"("Num In"=w2093) -> ("Meas Out"=w2095:T38[])  [unwired: 10 in]
                }
              }
            }
            n970 = call <vilib>:"Q.Enqueue Task.vi"("Top of Q"=TRUE, "Task Name"="Update Result Table", "Q In"=w2074) -> ()  [unwired: 7 in, 2 out]
            n971 = Bundle By Name(cluster=w2077, "Data.Meas"=w2071) -> (w2078:T73)
          }
          frame "Result - RTF Report" {
            n972 = Unbundle By Name(w2109) -> ("RptHdr"=w2121:T70, "RptUUT"=w2123:T50, "Data.Meas"=w2120:T38[], "ResultState"=w2114:T63)
            n973 = Unbundle By Name(w2114) -> ("Code"=w2113:i32, "Description"=w2112:string, "State"=w2111:T1)
            n974 = case shown="\"None\", Default" w2111 {
              tunnel: [TestResult.Symptom.State."Completed" ("Result.Result") TestResult.Symptom.State."Pass" ("Result.Result") TestResult.Symptom.State."Fail" ("Result.Result") TestResult.Symptom.State."Aborted" ("Result.Result") TestResult.Symptom.State."Error" ("Result.Result")] -> w2110
              frame "None", Default {
              }
              frame "Passing", "PASS" {
              }
              frame "Failing", "FAIL" {
              }
              frame "ABORT" {
              }
              frame "ERROR" {
              }
            }
            n975 = Bundle By Name(cluster=w2123, "Measurements.Measurement"=w2120, "Result.Code"=w2113, "Result.Description"=w2112, "Result.Result"=w2110) -> (w2116:T50)
            n976 = Unbundle By Name(w2107) -> ("Cfg.Dirs.Reports"=w2106:path)
            n977 = Build Path(base path=w2106, name or relative path="RTF") -> (appended path=w2104:path)
            n978 = Unbundle By Name(w2121) -> ("Station"=w2119:T47, "Test Run"=w2118:T48, "Test Sequence"=w2117:T49)  [unwired: 1 out]
            n979 = Build Array(w2116) -> (w2115:T50[])
            n980 = call <vilib>:"File.Create Folder if Does Not Exist.vi"("Path"=w2104) -> ("error out"=w2102:errorcluster, "Dup Path"=w2103:path)  [unwired: 8 in, 1 out]
            n981 = Bundle By Name(cluster=T46 {"#attributes"={"Version"="MTE_1.0.0"}, "Station"={"Name"="", "PN"="", "SN"="", "Rev"="", "PC Name"="", "Location"="", "HW_Config"={"HW_Item"=[]}, "SW_Config"={"SW_Item"=[]}}, "Test Run"={"Operator"="", "Start Time"=timestamp(0 s since 1904-01-01), "Duration(s)"=0.0, "Mode"="", "Comment"="", "ProcessStep"=""}, "Test Sequence"={"Name"="", "Config"={"Config_Item"=[]}}, "UUTs"={"UUT"=[]}} ("Test Result"), "Station"=w2119, "Test Run"=w2118, "Test Sequence"=w2117, "UUTs.UUT"=w2115) -> (w2108:T46)
            n982 = call "Result.Report Creator.vi"("error in"=w2102, "Data"=w2108, "Format"=Result.Report_Format_Selector."RTF", "OutputDir"=w2103) -> ("error out"=w2101:errorcluster, "Output File"=w2099:path)  [unwired: 6 in]
            n983 = call <vilib>:"File.Open File or Folder.vi"("Error In"=w2101, "Path"=w2099) -> ("Error Out"=w2100:errorcluster)  [unwired: 9 in]
          }
          frame "Result - Set Mode" {
            n984 = Variant To Data(type="", Variant=w2134) -> (data=w2132:string, error out=w2131:errorcluster)  [unwired: 1 in]
            n985 = case shown="No Error" w2131 {
              tunnel: w2136 -> [w2147 w2148]
              tunnel: [w2146 w2148] -> w2135
              tunnel: w2132 -> [w2142 _]
              tunnel: w2130 -> [w2145 _]
              frame No Error {
                n986 = Build Array("Mode", w2142) -> (w2141:string[])
                n987 = Build Array(w2141) -> (w2140:string[][])
                n988 = To Variant(anything=w2140) -> (Variant=w2139:variant)
                n989 = call <vilib>:"Q.Enqueue Task.vi"("Top of Q"=TRUE, "Data1"=w2139, "Task Name"="Set Variables", "Q In"=w2145) -> ()  [unwired: 6 in, 2 out]
                n990 = Bundle By Name(cluster=w2147, "RptHdr.Test Run.Mode"=w2142) -> (w2146:T73)
              }
              frame Error {
              }
            }
          }
          frame "Result - XML" {
            # "TODO - Add data files"
            n991 = Unbundle By Name(w2152) -> ("RptHdr"=w2164:T70, "RptUUT"=w2166:T50, "Data.Meas"=w2163:T38[], "ResultState"=w2157:T63)
            n992 = Unbundle By Name(w2157) -> ("Code"=w2156:i32, "Description"=w2155:string, "State"=w2154:T1)
            n993 = case shown="\"None\", Default" w2154 {
              tunnel: [TestResult.Symptom.State."Completed" ("Result.Result") TestResult.Symptom.State."Pass" ("Result.Result") TestResult.Symptom.State."Fail" ("Result.Result") TestResult.Symptom.State."Aborted" ("Result.Result") TestResult.Symptom.State."Error" ("Result.Result")] -> w2153
              frame "None", Default {
              }
              frame "Passing", "PASS" {
              }
              frame "Failing", "FAIL" {
              }
              frame "ABORT" {
              }
              frame "ERROR" {
              }
            }
            n994 = Unbundle By Name(w2149) -> ("Cfg.Dirs.Reports"=w2150:path)
            n995 = Bundle By Name(cluster=w2166, "Measurements.Measurement"=w2163, "Result.Code"=w2156, "Result.Description"=w2155, "Result.Result"=w2153) -> (w2159:T50)
            n996 = Unbundle By Name(w2164) -> ("Station"=w2162:T47, "Test Run"=w2161:T48, "Test Sequence"=w2160:T49)  [unwired: 1 out]
            n997 = Build Array(w2159) -> (w2158:T50[])
            n998 = Bundle By Name(cluster=T46 {"#attributes"={"Version"="MTE_1.0.0"}, "Station"={"Name"="", "PN"="", "SN"="", "Rev"="", "PC Name"="", "Location"="", "HW_Config"={"HW_Item"=[]}, "SW_Config"={"SW_Item"=[]}}, "Test Run"={"Operator"="", "Start Time"=timestamp(0 s since 1904-01-01), "Duration(s)"=0.0, "Mode"="", "Comment"="", "ProcessStep"=""}, "Test Sequence"={"Name"="", "Config"={"Config_Item"=[]}}, "UUTs"={"UUT"=[]}} ("Test Result"), "Station"=w2162, "Test Run"=w2161, "Test Sequence"=w2160, "UUTs.UUT"=w2158) -> (w2151:T46)
            n999 = call "Result.Report Creator.vi"("Data"=w2151, "Format"=Result.Report_Format_Selector."XML", "OutputDir"=w2150) -> ("error out"=w2167:errorcluster)  [unwired: 7 in, 1 out]
          }
          frame "Results - Overwrite Test Result State" {
            w2177 = T63 {"State"=enum."Passing", "Code"=0, "Description"=""}  # ResultState
            # "Result - Over Write Numeric Data(1D Array of Num Result)"
            n1000 = Variant To Data(type=w2177, Variant=w2182) -> (data=w2176:T63)  [unwired: 1 in, 1 out]
            n1001 = call <vilib>:"Q.Enqueue Task.vi"("Top of Q"=TRUE, "Task Name"="Update Result Table", "Q In"=w2178) -> ()  [unwired: 7 in, 2 out]
            n1002 = Unbundle By Name(w2175) -> ("ResultState.State"=w2174:T1)
            n1003 = case shown="Default" w2174 {
              tunnel: [w2184 w2187] -> w2181
              tunnel: w2176 -> [_ w2186]
              tunnel: w2175 -> [w2184 w2185]
              frame "ABORT" {
              }
              frame Default {
                n1004 = Bundle By Name(cluster=w2185, "ResultState"=w2186) -> (w2187:T73)
              }
            }
          }
          frame "Route Check" {
            n1005 = property on="Mode" class="Ring (strict)"() -> ("RingText.Text"=w2189:string)  [unwired: 2 in, 2 out]
            n1006 = Unbundle By Name(w2194) -> ("CfgFilePaths.WorkingCfg"=w2193:path)
            n1007 = local read "Station"() -> (w2192:T4)
            n1008 = Equal?(x="Engineering", y=w2189) -> (x = y?=w2188:bool)
            n1009 = Unbundle By Name(w2192) -> ("Name"=w2191:string)
            n1010 = call "TestExec.Route Check Dialog.vi"("Enable Maint"=w2188, "This Station's Name"=w2191, "Sta Config File"=w2193) -> ()  [unwired: 9 in]
          }
          frame "SeqCmd" {
            n1011 = Variant To Data(type="", Variant=w2204) -> (data=w2202:string)  [unwired: 1 in, 1 out]
            n1012 = Variant To Data(type=string[] [], Variant=w2207) -> (data=w2205:string[], error out=w2206:errorcluster)  [unwired: 1 in]
            n1013 = case shown="No Error" w2206 {
              selector: w2206 -> [w2209 _]
              tunnel: w2205 -> [w2211 _]
              tunnel: w2202 -> [w2213 w3679]
              tunnel: w2201 -> [w2216 w3684]
              tunnel: [w2215 w3684] -> w2200
              tunnel: w2199 -> [w2214 _]
              tunnel: w2198 -> [_ w3680]
              tunnel: [w2212 w3676] -> w2197
              tunnel: w2196 -> [w2210 _]
              frame No Error {
                n1014 = case shown="\"RunUtility\"" w2213 {
                  selector: w2213 -> [_ _ _ _ _ _ _ _ _ _ _ _ _ _ _ _ w2793 _ _ _ _ _ _ _ _ _ _ _ _ _ _ _ _ _ _ _ _ _ _ _ _ _ w3670]
                  tunnel: w2216 -> [w2221 w2255 w2268 w2309 w2351 w2386 w2430 w2451 w2489 w2526 w2542 w2558 w2581 w2633 w2732 w2758 w2788 w2871 w2897 w3026 w3035 w3207 w3224 w3243 w3257 w3273 w3380 w3394 w3435 w3446 w3469 w3479 w3500 w3522 w3572 w3590 w3603 w3609 w3622 w3628 w3658 w3660 w3675]
                  tunnel: [w2240 w2255 w2267 w2308 w2350 w2385 w2430 w2451 w2489 w2525 w2542 w2560 w2578 w2632 w2732 w2757 w2787 w2887 w2896 w3025 w3035 w3207 w3224 w3243 w3258 w3274 w3379 w3406 w3435 w3445 w3469 w3478 w3502 w3519 w3571 w3589 w3602 w3608 w3621 w3626 w3658 w3660 w3675] -> w2215
                  tunnel: w2214 -> [w2222 _ _ _ _ _ _ _ _ _ w2537 w2551 w2572 _ w2731 _ _ w2872 w2895 _ _ _ w3212 _ _ w3269 w3378 w3416 _ w3444 _ _ w3501 w3526 w3573 _ _ w3610 _ w3627 w3653 _ _]
                  tunnel: [_ _ _ _ _ _ _ _ w2477 _ _ w2565 w2584 w2629 _ _ w2785 _ _ _ _ _ w3217 _ _ _ _ _ _ _ _ _ _ _ _ _ _ _ _ _ _ _ w3669] -> w2212
                  tunnel: w2211 -> [w2223 w2254 w2270 w2311 w2353 w2384 w2426 w2453 w2490 w2527 w2536 _ w2585 w2631 w2719 w2756 w2792 w2873 w2892 w3033 w3037 _ w3223 w3248 w3266 w3270 w3377 w3417 w3429 w3442 _ w3477 w3499 w3535 w3570 w3588 w3601 w3607 _ w3629 w3652 w3659 _]
                  tunnel: w2210 -> [w2218 _ w2269 w2310 w2352 _ w2425 _ _ w2528 _ _ _ _ _ _ _ w2868 w2891 _ w3036 _ _ _ _ _ _ w3411 w3437 w3443 _ _ _ _ w3568 _ _ _ _ w3648 _ _ _]
                  tunnel: w2209 -> [_ _ _ _ _ _ _ _ _ _ _ _ _ w2630 _ _ _ _ w2893 _ _ _ _ _ _ _ _ _ _ _ _ _ _ _ _ _ _ _ _ _ _ _ _]
                  frame "Abort", "SetAbort" {
                    # "SetAbort(Desc)"
                    n1015 = Index Array(array=w2223) -> (element=w2237:string)  [unwired: 1 in]
                    n1016 = Unbundle By Name(w2221) -> ("Lists.Limits"=w2229:variant)
                    n1017 = Format Into String(format string="Test aborted by sequence: %s", w2237) -> (resulting string=w2236:string)  [unwired: 2 in, 1 out]
                    n1018 = Get Variant Attribute(Variant=w2229, name="CodePrefix", default value (empty Variant)=T25 {"Name"="", "LimType"=enum."None", "LL"="", "UL"="", "Units"="", "FailCode"=0, "FailDesc"=""} ("Result.Test Limit Item")) -> (value=w2231:T25)  [unwired: 1 in, 3 out]
                    n1019 = call <vilib>:"Q.Enqueue Task.vi"("Top of Q"=TRUE, "Task Name"="Sta Test Status", "Q In"=w2218) -> ()  [unwired: 7 in, 2 out]
                    n1020 = Unbundle By Name(w2231) -> ("FailCode"=w2227:i32)
                    n1021 = call "TestExec.Append Fault Code Prefix.vi"("Positive(F)\\Negative(T)"=TRUE ("Positive(F)\\Negative(T)"), "FaultCode"=-1 ("Code"), "FaultCode Prefix"=w2227) -> ("New Fault Code"=w2226:i32)  [unwired: 8 in]
                    n1022 = Bundle By Name(cluster=w2221, "ResultState.State"=SeqMgr.Result_State_Enum."ABORT" ("State"), "ResultState.Code"=w2226, "ResultState.Description"=w2236) -> (w2224:T73)
                    n1023 = Unbundle By Name(w2222) -> ("Log"=w2235:refnum<class "Event Notification.lvclass">)
                    n1024 = local write "Repeat Seq"(FALSE ("Repeat Seq")) -> ()
                    n1025 = call <vilib>:"Event Notification.Status Message.vi"("Log"=TRUE, "Level"=Event_Log.Log_Level."Verbose", "Message"=w2236, "Event Notification in"=w2235) -> ()  [unwired: 8 in]
                    n1026 = Unbundle By Name(w2224) -> ("SeqMgr"=w2243:refnum<class "SeqMgr.lvclass">)
                    n1027 = call <vilib>:"SeqMgr.Variables - Add, Replace.vi"("Name, Value"=string[][] [["Abort", "1"]] ("appended array"), "SeqMgr in"=w2243) -> ("SeqMgr out"=w2242:refnum<class "SeqMgr.lvclass">)  [unwired: 8 in, 1 out]
                    n1028 = Bundle By Name(cluster=w2224, "SeqMgr"=w2242) -> (w2240:T73)
                  }
                  frame "RepeatSequence" {
                    # "RepeatSequence(Enable,[Delay])"
                    n1029 = Index Array(array=w2254) -> (element #1=w2253:string, element #2=w2246:string)  [unwired: 2 in]
                    n1030 = Fract/Exp String To Number(string=w2246) -> (number=w2245:dbl)  [unwired: 3 in, 1 out]
                    n1031 = Equal?(x="1", y=w2253) -> (x = y?=w2248:bool)
                    n1032 = Empty String/Path?(string/path=w2246) -> (empty?=w2252:bool)
                    n1033 = Equal To 0?(x=w2245) -> (x = 0?=w2251:bool)
                    n1034 = Or(x=w2252, y=w2251) -> (x .or. y?=w2250:bool)
                    n1035 = Not(x=w2250) -> (.not. x?=w2249:bool)
                    n1036 = local write "Repeat Seq"(w2248) -> ()
                    n1037 = And(x=w2248, y=w2249) -> (x .and. y?=w2247:bool)
                    n1038 = case shown="True" w2247 {
                      tunnel: w2245 -> [_ w2256]
                      frame False {
                      }
                      frame True {
                        n1039 = local write "RepeatInt(s)"(w2256) -> ()
                      }
                    }
                  }
                  frame "Measurement" {
                    # "Measurement(Category, Name, Value,[Units, LimType, LL, UL, Status, Code, Description])"
                    n1040 = Index Array(array=w2270) -> (element #1=w2280:string, element #2=w2279:string, element #3=w2278:string, element #4=w2263:string, element #5=w2262:string, element #6=w2261:string, element #7=w2260:string, element #8=w2259:string, element #9=w2258:string, element #10=w2257:string)  [unwired: 10 in]
                    n1041 = call <vilib>:"Trim Whitespace.vi"("string"=w2259) -> ("trimmed string"=w2272:string)  [unwired: 1 in]
                    n1042 = case shown="\"FAIL\"" w2272 {
                      tunnel: [w2291 w2295 w2296 w2300] -> w2277
                      tunnel: w2258 -> [_ w2293 _ w2298]
                      tunnel: w2257 -> [_ w2294 _ w2299]
                      tunnel: [_ w2294 _ w2299] -> w2276
                      tunnel: [_ w2292 _ w2297] -> w2275
                      frame Default {
                        w2291 = T39 0 items=["LOG", "PASS", "FAIL", "ERROR"] ("Status")
                      }
                      frame "FAIL" {
                        w2295 = T39 2 items=["LOG", "PASS", "FAIL", "ERROR"] ("Status")
                        n1043 = Decimal String To Number(string=w2293) -> (number=w2292:i32)  [unwired: 2 in, 1 out]
                      }
                      frame "PASS" {
                        w2296 = T39 1 items=["LOG", "PASS", "FAIL", "ERROR"] ("Status")
                      }
                      frame "ERROR" {
                        w2300 = T39 3 items=["LOG", "PASS", "FAIL", "ERROR"] ("Status")
                        n1044 = Decimal String To Number(string=w2298) -> (number=w2297:i32)  [unwired: 2 in, 1 out]
                      }
                    }
                    n1045 = call <vilib>:"Q.Enqueue Task.vi"("Top of Q"=TRUE, "Task Name"="Update Result Table", "Q In"=w2269) -> ()  [unwired: 7 in, 2 out]
                    n1046 = Unbundle By Name(w2268) -> ("ResultState"=w2284:T63, "SectCtr"=w2290:T72, "Data.Meas"=w2287:T38[], "Lists.Limits"=w2264:variant)
                    n1047 = Bundle By Name(cluster=T38 {"Cnt"=0, "Step"="", "Category"="", "Name"="", "Value"="", "Units"="", "LimType"="", "LL"="", "UL"="", "Status"=0, "Code"=0, "Desc"="", "Time"=timestamp(0 s since 1904-01-01)} ("Meas"), "Category"=w2280, "Name"=w2279, "Value"=w2278, "Units"=w2263, "LimType"=w2262, "LL"=w2261, "UL"=w2260, "Status"=w2277, "Code"=w2275, "Desc"=w2276) -> (w2266:T38)
                    n1048 = call "Result.Measurement Look Up Limits.vi"("Meas"=w2266, "Limits"=w2264) -> ("Measurement Out"=w2265:T38)  [unwired: 4 in]
                    n1049 = call "Step Counter.Step Count Controller.vi"("Step Action"=Step_Counter.Action."Data +", "Step State"=w2290) -> ("Step"=w2283:string, "Step State Out"=w2289:T72, "Cntr"=w2271:i32)  [unwired: 7 in]
                    n1050 = Bundle By Name(cluster=w2265, "Step"=w2283, "Cnt"=w2271) -> (w2288:T38)
                    n1051 = Build Array (concatenate)(w2287, w2288) -> (w2285:T38[])
                    n1052 = call "Result.Measurement, Screen for Fail or Error.vi"("Num"=w2285, "ResultState In"=w2284) -> ("ResultState Out"=w2286:T63)  [unwired: 9 in]
                    n1053 = Bundle By Name(cluster=w2268, "ResultState"=w2286, "SectCtr"=w2289, "Data.Meas"=w2285) -> (w2267:T73)
                  }
                  frame "AddAttribute", "AddAttributeResult" {
                    w2301 = "" ("Units")
                    # "Measurement(Category, Name, Value,[Units, LimType, LL, UL, Status, Code, Description])"
                    n1054 = Index Array(array=w2311) -> (element #1=w2321:string, element #2=w2320:string, element #3=w2319:string, element #4=w2304:string, element #5=w2303:string, element #6=w2302:string)  [unwired: 6 in]
                    n1055 = call <vilib>:"Trim Whitespace.vi"("string"=w2304) -> ("trimmed string"=w2313:string)  [unwired: 1 in]
                    n1056 = case shown="\"FAIL\"" w2313 {
                      tunnel: [w2332 w2336 w2337 w2341] -> w2318
                      tunnel: w2303 -> [_ w2334 _ w2339]
                      tunnel: w2302 -> [_ w2335 _ w2340]
                      tunnel: [_ w2335 _ w2340] -> w2317
                      tunnel: [_ w2333 _ w2338] -> w2316
                      frame Default {
                        w2332 = T39 0 items=["LOG", "PASS", "FAIL", "ERROR"] ("Status")
                      }
                      frame "FAIL" {
                        w2336 = T39 2 items=["LOG", "PASS", "FAIL", "ERROR"] ("Status")
                        n1057 = Decimal String To Number(string=w2334) -> (number=w2333:i32)  [unwired: 2 in, 1 out]
                      }
                      frame "PASS" {
                        w2337 = T39 1 items=["LOG", "PASS", "FAIL", "ERROR"] ("Status")
                      }
                      frame "ERROR" {
                        w2341 = T39 3 items=["LOG", "PASS", "FAIL", "ERROR"] ("Status")
                        n1058 = Decimal String To Number(string=w2339) -> (number=w2338:i32)  [unwired: 2 in, 1 out]
                      }
                    }
                    n1059 = call <vilib>:"Q.Enqueue Task.vi"("Top of Q"=TRUE, "Task Name"="Update Result Table", "Q In"=w2310) -> ()  [unwired: 7 in, 2 out]
                    n1060 = Unbundle By Name(w2309) -> ("ResultState"=w2325:T63, "SectCtr"=w2331:T72, "Data.Meas"=w2328:T38[], "Lists.Limits"=w2305:variant)
                    n1061 = Bundle By Name(cluster=T38 {"Cnt"=0, "Step"="", "Category"="", "Name"="", "Value"="", "Units"="", "LimType"="", "LL"="", "UL"="", "Status"=0, "Code"=0, "Desc"="", "Time"=timestamp(0 s since 1904-01-01)} ("Meas"), "Category"=w2321, "Name"=w2320, "Value"=w2319, "Units"=w2301, "LimType"=w2301, "LL"=w2301, "UL"=w2301, "Status"=w2318, "Code"=w2316, "Desc"=w2317) -> (w2307:T38)
                    n1062 = call "Result.Measurement Look Up Limits.vi"("Meas"=w2307, "Limits"=w2305) -> ("Measurement Out"=w2306:T38)  [unwired: 4 in]
                    n1063 = call "Step Counter.Step Count Controller.vi"("Step Action"=Step_Counter.Action."Data +", "Step State"=w2331) -> ("Step"=w2324:string, "Step State Out"=w2330:T72, "Cntr"=w2312:i32)  [unwired: 7 in]
                    n1064 = Bundle By Name(cluster=w2306, "Step"=w2324, "Cnt"=w2312) -> (w2329:T38)
                    n1065 = Build Array (concatenate)(w2328, w2329) -> (w2326:T38[])
                    n1066 = call "Result.Measurement, Screen for Fail or Error.vi"("Num"=w2326, "ResultState In"=w2325) -> ("ResultState Out"=w2327:T63)  [unwired: 9 in]
                    n1067 = Bundle By Name(cluster=w2309, "ResultState"=w2327, "SectCtr"=w2330, "Data.Meas"=w2326) -> (w2308:T73)
                  }
                  frame "AddNumericResult" {
                    w2346 = "" ("Units")
                    # "Cmd_AddNumericResult(Category,Name,Value,Units,Result,[Code,Desc])"
                    n1068 = Index Array(array=w2353) -> (element #1=w2363:string, element #2=w2362:string, element #3=w2361:string, element #4=w2342:string, element #5=w2343:string, element #6=w2344:string, element #7=w2345:string)  [unwired: 7 in]
                    n1069 = call <vilib>:"Trim Whitespace.vi"("string"=w2343) -> ("trimmed string"=w2355:string)  [unwired: 1 in]
                    n1070 = case shown="\"FAIL\"" w2355 {
                      tunnel: [w2374 w2378 w2379 w2383] -> w2360
                      tunnel: w2344 -> [_ w2376 _ w2381]
                      tunnel: w2345 -> [_ w2377 _ w2382]
                      tunnel: [_ w2377 _ w2382] -> w2359
                      tunnel: [_ w2375 _ w2380] -> w2358
                      frame Default {
                        w2374 = T39 0 items=["LOG", "PASS", "FAIL", "ERROR"] ("Status")
                      }
                      frame "FAIL" {
                        w2378 = T39 2 items=["LOG", "PASS", "FAIL", "ERROR"] ("Status")
                        n1071 = Decimal String To Number(string=w2376) -> (number=w2375:i32)  [unwired: 2 in, 1 out]
                      }
                      frame "PASS" {
                        w2379 = T39 1 items=["LOG", "PASS", "FAIL", "ERROR"] ("Status")
                      }
                      frame "ERROR" {
                        w2383 = T39 3 items=["LOG", "PASS", "FAIL", "ERROR"] ("Status")
                        n1072 = Decimal String To Number(string=w2381) -> (number=w2380:i32)  [unwired: 2 in, 1 out]
                      }
                    }
                    n1073 = call <vilib>:"Q.Enqueue Task.vi"("Top of Q"=TRUE, "Task Name"="Update Result Table", "Q In"=w2352) -> ()  [unwired: 7 in, 2 out]
                    n1074 = Unbundle By Name(w2351) -> ("ResultState"=w2367:T63, "SectCtr"=w2373:T72, "Data.Meas"=w2370:T38[], "Lists.Limits"=w2347:variant)
                    n1075 = Bundle By Name(cluster=T38 {"Cnt"=0, "Step"="", "Category"="", "Name"="", "Value"="", "Units"="", "LimType"="", "LL"="", "UL"="", "Status"=0, "Code"=0, "Desc"="", "Time"=timestamp(0 s since 1904-01-01)} ("Meas"), "Category"=w2363, "Name"=w2362, "Value"=w2361, "Units"=w2342, "LimType"=w2346, "LL"=w2346, "UL"=w2346, "Status"=w2360, "Code"=w2358, "Desc"=w2359) -> (w2349:T38)
                    n1076 = call "Result.Measurement Look Up Limits.vi"("Meas"=w2349, "Limits"=w2347) -> ("Measurement Out"=w2348:T38)  [unwired: 4 in]
                    n1077 = call "Step Counter.Step Count Controller.vi"("Step Action"=Step_Counter.Action."Data +", "Step State"=w2373) -> ("Step"=w2366:string, "Step State Out"=w2372:T72, "Cntr"=w2354:i32)  [unwired: 7 in]
                    n1078 = Bundle By Name(cluster=w2348, "Step"=w2366, "Cnt"=w2354) -> (w2371:T38)
                    n1079 = Build Array (concatenate)(w2370, w2371) -> (w2368:T38[])
                    n1080 = call "Result.Measurement, Screen for Fail or Error.vi"("Num"=w2368, "ResultState In"=w2367) -> ("ResultState Out"=w2369:T63)  [unwired: 9 in]
                    n1081 = Bundle By Name(cluster=w2351, "ResultState"=w2369, "SectCtr"=w2372, "Data.Meas"=w2368) -> (w2350:T73)
                  }
                  frame "AddEquipmentItem" {
                    # "AddEquipmentItem(Name,Mfg,PN,SN,SW_FW,Note)"
                    n1082 = Index Array(array=w2384) -> (element #1=w2392:string, element #2=w2399:string, element #3=w2398:string, element #4=w2397:string, element #5=w2396:string, element #6=w2395:string)  [unwired: 6 in]
                    n1083 = Unbundle By Name(w2386) -> ("RptHdr.Station.HW_Config.HW_Item"=w2393:T41[])
                    n1084 = Bundle By Name(cluster=T41 {"Name"="", "MFG"="", "PN"="", "SN"="", "SW/FW"="", "Note"="", "Cal_ID"="", "Cal_Type"="", "Cal_Due_Date"=timestamp(0 s since 1904-01-01), "Cal_Status"=""} ("Hardware Item"), "Name"=w2392, "MFG"=w2399, "PN"=w2398, "SN"=w2397, "SW/FW"=w2396, "Note"=w2395) -> (w2394:T41)
                    n1085 = for {
                      tunnel: w2393 -> [w2404] mode=indexing
                      tunnel: w2392 -> [w2402]
                      tunnel: [w2401] -> w2391
                      tunnel: [w2400] -> w2390
                      i -> [w2400]
                      stop <- w2401 stop-if-true
                      n1086 = Unbundle By Name(w2404) -> ("Name"=w2403:string)
                      n1087 = Equal?(x=w2403, y=w2402) -> (x = y?=w2401:bool)
                    }
                    n1088 = case shown="True" w2391 {
                      tunnel: w2393 -> [w2407 w2411]
                      tunnel: [w2406 w2408] -> w2389
                      tunnel: w2394 -> [w2405 w2409]
                      tunnel: w2390 -> [_ w2410]
                      frame False {
                        n1089 = Build Array (concatenate)(w2407, w2405) -> (w2406:T41[])
                      }
                      frame True {
                        n1090 = Replace Array Subset(array=w2411, new element=w2409, index=w2410) -> (w2408:T41[])
                      }
                    }
                    n1091 = Bundle By Name(cluster=w2386, "RptHdr.Station.HW_Config.HW_Item"=w2389) -> (w2385:T73)
                    n1092 = call "TestExec.Eq List to Table.vi"("Eq List"=w2389) -> ("Table"=w2388:string[][])
                    n1093 = local write "Equipment List"(w2388) -> ()
                  }
                  frame "AddResultDataFile" {
                    # "AddResultDataFile(Folder,FileName, Category,Name)"
                    n1094 = Index Array(array=w2426) -> (element #1=w2429:string, element #2=w2427:string, element #3=w2422:string, element #4=w2423:string)  [unwired: 4 in]
                    n1095 = call <vilib>:"Trim Whitespace.vi"("string"=w2427) -> ("trimmed string"=w2415:string)  [unwired: 1 in]
                    n1096 = call <vilib>:"File.Remove Name Extension.vi"("File Name"=w2415) -> ("Ext"=w2416:string, "Name Less Ext"=w2417:string)  [unwired: 1 in]
                    n1097 = String To Path(string=w2429) -> (path=w2428:path)
                    n1098 = Build Path(base path=w2428, name or relative path=w2415) -> (appended path=w2421:path)
                    n1099 = case shown="Default" w2423 {
                      selector: w2423 -> [w2433 _]
                      tunnel: [w2433 w2434] -> w2418
                      tunnel: w2417 -> [_ w2434]
                      frame Default {
                      }
                      frame "" {
                      }
                    }
                    n1100 = case shown="Default" w2422 {
                      selector: w2422 -> [w2431 _]
                      tunnel: [w2431 "File"] -> w2419
                      frame Default {
                      }
                      frame "" {
                      }
                    }
                    n1101 = Get Date/Time In Seconds() -> (seconds since 1Jan1904=w2412:timestamp)
                    n1102 = call "Time.TimeStamp to String.vi"("Time Stamp in"=w2412) -> ("Time String Out"=w2420:string)  [unwired: 10 in]
                    n1103 = Bundle By Name(cluster=T29 {"Cnt"=0, "Step"="", "Category"="", "Name"="", "Type"="", "File Name"="", "Time"="", "Path"=path ""} ("FileData Object"), "Time"=w2420, "Path"=w2421, "File Name"=w2415, "Type"=w2416, "Category"=w2419, "Name"=w2418) -> (w2414:T29)
                    n1104 = Build Array(w2414) -> (w2413:T29[])
                    n1105 = call "TestExec.Result, File Data Objs.vi"("File Data Objs"=w2413, "Q In"=w2425) -> ()  [unwired: 9 in, 1 out]
                  }
                  frame "ArchiveUUTData" {
                    n1106 = Unbundle By Name(w2451) -> ("UUT Dir"=w2440:path, "CfgFilePaths.Archive"=w2450:path, "ResultState.State"=w2449:T1, "ResultState.Code"=w2437:i32)
